vi "PH_Beamline_Chief.PC Set Settings.vi"(0 "VI in":refnum<vi>, 2 "Settings":T1, 5 "error in (no error)":errorcluster) -> (14 "VI out":refnum<vi>, 19 "error out":errorcluster)   [LabVIEW 2014, in "PH_Beamline_Chief.lvlib"]
uses:
  PH_Beamline_Chief.lvlib
  PH_Beamline_Chief.Settings.ctl
  lib.lib/DimLVEvent/LVDimInterface/LVDimInterface.lvlib
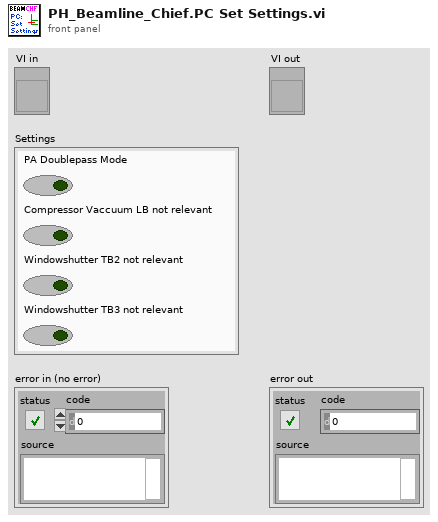
[diagram p1: front panel]
types:
  T1 = typedef "PH_Beamline_Chief.lvlib/PH_Beamline_Chief.Settings.ctl" = cluster{"PA Doublepass Mode":bool, "Compressor Vaccuum LB not relevant":bool, "Windowshutter TB2 not relevant":bool, "Windowshutter TB3 not relevant":bool}
  T2 = typedef "PH_Beamline_Chief.lvlib/PH_Beamline_Chief.i attribute.ctl" = cluster{"BL Service IDs":cluster{"YLF_BL_Status":i32, "fs_BL_Status":i32, "fs_YLF_BL_Status":i32, "ns_BL_Status":i32, "PA_Input_BL_Status":i32, "PA_UnDelay_BL_Status":i32, "PA_Delay_BL_Status":i32, "PA_BL_Status":i32, "PA_Bypass_BL_Status":i32, "PA_Exit_BL_Status":i32, "PA_LL_BL_Status":i32, "LL_BL_Status":i32, "PA_MA_BL_Status":i32, "MA_Exit_BL_Status":i32, "MA_Z6_BL_Status":i32, "Z6_BL_Status":i32, "MA_LB_BL_Status":i32, "LB_TB2_BL_Status":i32, "PA_before_Bypass_BL_Status":i32, "LB_TB3_BL_Status":i32}, "R2S Service ID":i32, "Settings":cluster{"Wanted":T1, "GUI Ref":refnum<vi>, "Service ID":i32}}
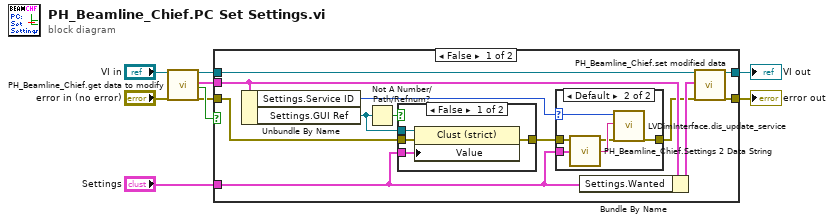
[diagram p0: block diagram]
diagram:
  n1 = call "PH_Beamline_Chief.get data to modify.vi"("i ref in"="VI in", "error in (no error)"="error in (no error)") -> ("i ref out"=w2:refnum<vi>, "i attribute"=w7:T2, "timed out"=w9:bool, "error out"=w4:errorcluster)  [unwired: 14 in]
  n2 = case shown="False" w9 {
    tunnel: w2 -> [w21 w34]
    tunnel: w4 -> [w20 w33]
    tunnel: [w19 w34] -> w5
    tunnel: [w18 w33] -> w6
    tunnel: w7 -> [w16 _]
    tunnel: "Settings" -> [w11 _]
    frame False {
      n3 = Unbundle By Name(w16) -> ("Settings.Service ID"=w10:i32, "Settings.GUI Ref"=w14:refnum<vi>)
      n4 = Not A Number/Path/Refnum?(number/path/refnum=w14) -> (NaN/Path/Refnum?=w15:bool)
      n5 = case shown="False" w15 {
        tunnel: w20 -> [w31 w32]
        tunnel: [w30 w32] -> w13
        tunnel: w14 -> [w29 _]
        tunnel: w11 -> [w28 _]
        frame False {
          n6 = property class="Clust (strict)"(reference=w29, error in=w31, "Value"=w28) -> (error out=w30:errorcluster)  [unwired: 1 out]
        }
        frame True {
        }
      }
      n7 = case shown="Default" w10 {
        selector: w10 -> [_ w24]
        tunnel: [w22 w27] -> w12
        tunnel: w11 -> [_ w26]
        tunnel: w13 -> [w22 w23]
        frame -1 {
        }
        frame Default {
          n8 = call "PH_Beamline_Chief.Settings 2 Data String.vi"("Settings"=w26) -> ("Data String"=w25:string)
          n9 = call "LVDimInterface.dis_update_service.vi"("my_serviceID"=w24, "data"=w25, "error in (no error)"=w23) -> ("error out"=w27:errorcluster)  [unwired: 14 in, 2 out]
        }
      }
      n10 = Bundle By Name(cluster=w16, "Settings.Wanted"=w11) -> (w17:T2)
      n11 = call "PH_Beamline_Chief.set modified data.vi"("i ref in"=w21, "i attribute"=w17, "error in (no error)"=w12) -> ("i ref out"=w19:refnum<vi>, "error out"=w18:errorcluster)  [unwired: 15 in]
    }
    frame True {
    }
  }
  "error out" <- w6
  "VI out" <- w5
